vi "UMLEditor Main.vi"(1 "StartProject":string, 3 "StartTarget":string) -> ()   [LabVIEW 2012] (continued)
          n2182 = call-dynamic "getClassInfo.vi"("reference"=w5675, "error in (no error)"=w5689) -> ("reference out"=w5688:refnum<class "ClassNode.lvclass">, "className"=w5685:string, "ClassPath"=w5686:path, "error out"=w5687:errorcluster)  [unwired: 8 in, 6 out]
          n2183 = Select(t=-1, s=w5673, f=w5670) -> (s? t:f=w5672:i32)
          n2184 = Empty String/Path?(string/path=w5686) -> (empty?=w5694:bool)
          n2185 = Not A Number/Path/Refnum?(number/path/refnum=w5686) -> (NaN/Path/Refnum?=w5693:bool)
          n2186 = Or(x=w5694, y=w5693) -> ()  [unwired: 1 out]
          n2187 = Increment(x=w5670) -> (x+1=w5667:i32)
          n2188 = call <resource>:"ReversedEngineering SyncUmlFromCode.vi"("SyncAction"=ReversedEngineering_SyncUmlFromCodeActions."GetAll", "ClassPath"=w5686, "NodeRef"=w5688, "GraphRef"=w5692, "IgnoreClasses"=w5678, "error in (no error)"=w5687, "ClassName(needed for lllbs)"=w5685, "graphics"=w5691, "IterationNo"=w5672, "grid"=w5690, "IterationsN"=w5666) -> ("Cancelled"=w5674:bool, "ClassName"=w5680:string, "attributes"=w5682:string, "methods"=w5681:string, "error out"=w5683:errorcluster)  [unwired: 1 in, 3 out]
          n2189 = Empty String/Path?(string/path=w5680) -> (empty?=w5679:bool)
          n2190 = case shown="False" w5679 {
            tunnel: w5683 -> [w5704 w5709]
            tunnel: w5682 -> [w5703 _]
            tunnel: w5681 -> [w5702 _]
            tunnel: [w5698 w5709] -> w5695
            tunnel: w5688 -> [w5697 _]
            tunnel: w5680 -> [w5696 _]
            frame False {
              n2191 = call-dynamic "ExternalSetParam.vi"("reference"=w5697, "setParameter"=ExternalSetTypes."Attributes", "string"=w5703, "error in (no error)"=w5704) -> ("reference out"=w5706:refnum<class "ClassNode.lvclass">, "error out"=w5707:errorcluster)  [unwired: 14 in]
              n2192 = call-dynamic "ExternalSetParam.vi"("reference"=w5706, "setParameter"=ExternalSetTypes."Methods", "string"=w5702, "error in (no error)"=w5707) -> ("reference out"=w5699:refnum<class "ClassNode.lvclass">, "error out"=w5700:errorcluster)  [unwired: 14 in]
              n2193 = call-dynamic "ExternalSetParam.vi"("reference"=w5699, "setParameter"=ExternalSetTypes."Name", "string"=w5696, "error in (no error)"=w5700) -> ("error out"=w5698:errorcluster)  [unwired: 14 in, 1 out]
            }
            frame True {
            }
          }
          n2194 = Format Into String(format string="Synchronizing %d of %d", w5667, w5666) -> (resulting string=w5668:string)  [unwired: 2 in, 1 out]
          n2195 = local write "StatusBar"(w5668) -> ()
        }
        n2196 = case shown="True" w5635 {
          tunnel: w5634 -> [_ _]
          tunnel: w5632 -> [w5658 w5661]
          tunnel: [w5658 w5660] -> w5631
          frame False {
          }
          frame True {
            n2197 = Get Date/Time In Seconds() -> (seconds since 1Jan1904=w5659:timestamp)
            n2198 = Bundle By Name(cluster=w5661, "LastSync"=w5659) -> (w5660:T7)
            n2199 = property on="Picture" class="Pict"("DisabledEnum"=T38."Enabled" ("Disabled")) -> (error out=w5662:errorcluster)  [unwired: 2 in, 1 out]
            n2200 = call <vilib>:"Unset Busy.vi"("error in (no error)"=w5662) -> ()  [unwired: 10 in, 1 out]
          }
        }
        n2201 = stacked-sequence {
          tunnel: w5634 -> [_]
          tunnel: w5633 -> [w5657]
          frame #0 {
            n2202 = local write "StatusBar"(w5657) -> ()
          }
        }
        n2203 = call <resource>:"UMLEditor setDiagramInfo.vi"("error in (no error)"=w5634, "localVariablesIn"=w5631, "action"=enum16{"Name/Dir", "Unsaved", "Saved"}."Unsaved") -> ("localVariablesOut"=w5646:T7, "error out"=w5648:errorcluster)  [unwired: 2 in, 13 out]
        n2204 = call-dynamic "layout.vi"("reference"=w5642, "error in (no error)"=w5648) -> ("error out"=w5643:errorcluster)  [unwired: 16 in, 1 out]
      }
      frame "StraightenAssociation" {
        n2205 = call <resource>:"UMLEditor getDiagramInfo.vi"("localVariables"=w5727, "error in (no error)"=w5735) -> ("graph"=w5734:refnum<class "Graph.lvclass">, "error out"=w5730:errorcluster)  [unwired: 16 out]
        n2206 = call-dynamic "getEdges.vi"("reference"=w5734, "error in (no error)"=w5730) -> ("reference out"=w5726:refnum<class "Graph.lvclass">, "edges"=w5729:refnum<class "AbstractEdge.lvclass">[], "error out"=w5728:errorcluster)  [unwired: 15 in]
        n2207 = Unbundle By Name(w5727) -> ("graphics"=w5725:refnum<class "Graphics.lvclass">, "grid"=w5724:refnum<class "Grid.lvclass">)
        n2208 = for {
          shift-right: [w5741] -> w5732
          shift-left: w5728 -> [w5744]
          tunnel: w5729 -> [w5743] mode=indexing
          tunnel: w5726 -> [w5739]
          tunnel: w5725 -> [w5738]
          tunnel: w5724 -> [w5737]
          n2209 = call-dynamic "StraightenAssociations.vi"("reference"=w5743, "error in (no error)"=w5744) -> ("reference out"=w5740:refnum<class "AbstractEdge.lvclass">, "error out"=w5742:errorcluster)  [unwired: 16 in]
          n2210 = call-dynamic "Layout.vi"("reference"=w5740, "graph"=w5739, "graphics"=w5738, "grid"=w5737, "error in (no error)"=w5742) -> ("error out"=w5741:errorcluster)  [unwired: 13 in, 1 out]
        }
        n2211 = call <resource>:"UMLEditor setDiagramInfo.vi"("error in (no error)"=w5732, "localVariablesIn"=w5727, "action"=enum16{"Name/Dir", "Unsaved", "Saved"}."Unsaved") -> ("localVariablesOut"=w5731:T7, "error out"=w5723:errorcluster)  [unwired: 2 in, 13 out]
      }
      frame "Exit" {
        # "Check if any unsaved"
        n2212 = Unbundle By Name(w5751) -> ("diagrams"=w5755:T39)
        n2213 = for {
          tunnel: w5755 -> [w5765] mode=indexing
          tunnel: [w5764] -> w5754 mode=indexing
          n2214 = Unbundle By Name(w5765) -> ("unsaved"=w5764:bool)
        }
        n2215 = local read "toolTab"() -> (w5747:enum32{"Class", "Sequence", "UseCase", "State"})
        n2216 = Search 1D Array(1D array=w5754, element=TRUE) -> (index of element=w5750:i32)  [unwired: 1 out]
        n2217 = case shown="\"Class\", Default" w5747 {
          tunnel: [diagramType."Sequency" ("diagramType") diagramType."UseCase" ("diagramType") diagramType."State" ("diagramType") diagramType."Class" ("diagramType")] -> w5746
          frame "Sequence" {
          }
          frame "UseCase" {
          }
          frame "State" {
          }
          frame "Class", Default {
          }
        }
        n2218 = Bundle By Name(cluster=w5751, "quit"=TRUE ("element"), "diagramIndex"=w5750) -> (w5752:T7)
        n2219 = Greater Or Equal To 0?(x=w5750) -> (x >= 0?=w5749:bool)
        n2220 = Select(t=UMLEditor_statesType."Close" ("state"), s=w5749, f=UMLEditor_statesType."QUIT") -> (s? t:f=w5758:T8)
        n2221 = case shown="\"QUIT\"" w5758 {
          tunnel: [w5766 w5769] -> w5759
          tunnel: w5745 -> [w5766 w5773]
          tunnel: w5752 -> [_ w5772]
          tunnel: w5746 -> [_ w5768]
          frame "Idle", Default {
          }
          frame "QUIT" {
            n2222 = call <resource>:"UMLEditor saveIniFileInfo.vi"("localVariables"=w5772, "error in (no error)"=w5773, "diagramType"=w5768) -> ("error out"=w5770:errorcluster)  [unwired: 16 out]
            n2223 = Unbundle By Name(w5770) -> ("code"=w5771:i32)
            n2224 = call <resource>:"UMLEditor_IniFilePath.vi"() -> ("Get Path"=w5767:path)  [unwired: 2 in, 17 out]
            n2225 = case shown="7, 8" w5771 {
              tunnel: w5770 -> [w5774 _]
              tunnel: [w5774 errorcluster {"status"=FALSE, "code"=0, "source"=""} ("error out")] -> w5769
              tunnel: w5767 -> [_ w5775]
              frame 0, Default {
              }
              frame 7, 8 {
                n2226 = Format Into String(format string="File permission error.\n\nMake sure the file to modify is writable.\n%s" ("message"), w5775) -> (resulting string=w5777:string)  [unwired: 2 in, 1 out]
                n2227 = One Button Dialog(message=w5777) -> ()  [unwired: 2 out]
              }
            }
          }
        }
      }
      frame "Error", Default {
        n2228 = Format Into String(w5782) -> (resulting string=w5781:string)  [unwired: 3 in, 1 out]
        n2229 = Unbundle By Name(w5779) -> ("code"=w5784:i32)
        n2230 = case shown="1055" w5784 {
          tunnel: [TRUE ("s") FALSE ("s") FALSE ("s") FALSE ("s") FALSE ("s") FALSE ("s") FALSE ("s") FALSE ("s") FALSE ("s") _ FALSE ("s")] -> w5783
          tunnel: w5781 -> [w5791 _ _ _ _ _ _ _ _ _ _]
          tunnel: w5780 -> [w5790 _ _ _ _ _ _ _ _ _ _]
          tunnel: w5779 -> [_ _ _ _ _ _ _ _ _ w5809 _]
          frame 0, Default {
            n2231 = call <resource>:"GDSError_LogErrorInformation.vi"("State"=w5791, "LocalVariableData"=w5790) -> ()  [unwired: 2 in, 16 out]
          }
          frame 1106, 1108 {
            n2232 = One Button Dialog(message="The saved file you tried to open,\nwas not compatible with this version.") -> ()  [unwired: 2 out]
          }
          frame 1044 {
            n2233 = One Button Dialog(message="A VI was locked, so the task has been stopped.") -> ()  [unwired: 2 out]
          }
          frame 1073 {
            n2234 = One Button Dialog(message="Trying to access a write protected file, or\na file that is currently running or reserved\nfor execution.") -> ()  [unwired: 2 out]
          }
          frame 56003 {
            n2235 = One Button Dialog(message="The new class(es) could not be added to the project since it would cause a conflict with an item already in memory.\n-This could be due to that the class created already exists in another opened project. Try to close other none used project to prevent this from happening.") -> ()  [unwired: 2 out]
          }
          frame 1025 {
            n2236 = One Button Dialog(message="The project reference is invalid.\nMake sure you have a selected project.") -> ()  [unwired: 2 out]
          }
          frame 1055 {
            n2237 = One Button Dialog(message="Class/Project reference error.\nThe reason for this could be:\n-The project has been closed\n-The class(es) has been removed from the project\n-The class(es) don't exist in the selected project") -> ()  [unwired: 2 out]
          }
          frame 7000 {
            n2238 = One Button Dialog(message="The class reference could not be obtained from the project.\nThe reason for this could be:\n-The project has been closed\n-The class has been removed from the project\n-The class don't exist in the selected project") -> ()  [unwired: 2 out]
          }
          frame 56001 {
            n2239 = One Button Dialog(message="Class(es) with the same name already exists in the project.") -> ()  [unwired: 2 out]
          }
          frame 5011 {
            n2240 = call <resource>:"GDSError_ReportError.vi"("error in (no error)"=w5809) -> ()  [unwired: 19 out]
          }
          frame 8 {
            n2241 = One Button Dialog(message="File permission error.\n\nMake sure the file to modify is writable.") -> ()  [unwired: 2 out]
          }
        }
        n2242 = Select(t=w5779, s=w5783, f=errorcluster {"status"=FALSE, "code"=0, "source"=""} ("error out")) -> (s? t:f=w5785:errorcluster)
        n2243 = Select(t=UMLEditor_statesType."QUIT" ("state"), s=w5783, f=UMLEditor_statesType."Idle" ("state")) -> (s? t:f=w5789:T8)
      }
    }
    n2244 = Select(t=UMLEditor_statesType."Error" ("state"), s=w32, f=w37) -> (s? t:f=w38:T8)
    n2245 = case shown="Error" w32 {
      frame No Error {
      }
      frame Error {
      }
    }
    n2246 = Equal?(x=w37, y=UMLEditor_statesType."QUIT" ("state")) -> (x = y?=w45:bool)
  }
  n2247 = Unbundle By Name(w9) -> ("graphics"=w24:refnum<class "Graphics.lvclass">, "grid"=w26:refnum<class "Grid.lvclass">, "diagrams"=w22:T39)
  n2248 = for {
    shift-right: [w5813] -> w23
    shift-left: w5 -> [w5814]
    tunnel: w22 -> [w5815] mode=indexing
    n2249 = Unbundle By Name(w5815) -> ("graph"=w5812:refnum<class "Graph.lvclass">)
    n2250 = call-dynamic "Destroy.vi"("reference"=w5812, "error in (no error)"=w5814) -> ("error out"=w5813:errorcluster)  [unwired: 16 in, 1 out]
  }
  n2251 = call-dynamic "Destroy.vi"("reference"=w26, "error in (no error)"=w23) -> ("error out"=w25:errorcluster)  [unwired: 16 in, 1 out]
  n2252 = call-dynamic "Destroy.vi"("reference"=w24, "error in (no error)"=w25) -> ("# of objects"=w12:i32)  [unwired: 16 in, 1 out]
  n2253 = case shown="Error" w5 {
    selector: w5 -> [w5816 w5817]
    tunnel: [w5816 w5817] -> w20
    tunnel: w9 -> [_ _]
    tunnel: w12 -> [_ _]
    frame No Error {
    }
    frame Error {
      n2254 = call <resource>:"GDSError_ReportError.vi"("error in (no error)"=w5817) -> ()  [unwired: 19 out]
    }
  }
  n2255 = Unbundle By Name(w9) -> ("Cursors"=w4:refnum<k1>[])
  n2256 = Unbundle By Name(w9) -> ("Event"=w8:refnum<event-registration>, "ViRef"=w19:refnum<vi>)
  n2257 = Close Reference(reference=w19, error in (no error)=w20) -> (error out=w17:errorcluster)
  n2258 = stacked-sequence {
    tunnel: w17 -> [w5826]
    tunnel: [w5826] -> w16
    tunnel: w8 -> [w5819]
    tunnel: w4 -> [w5818]
    frame #0 {
      # "Kill Tasks"
      n2259 = call <resource>:"ContextHelp_StopPopUpTask.vi"() -> ()  [unwired: 2 in, 18 out]
      n2260 = call <resource>:"UMLEditor ClipBoard.vi"("menuAction"=UMLEditor_ClipBoardActionType."EmptyClipBoard") -> ()  [unwired: 5 in, 14 out]
      n2261 = call <resource>:"CleanUp.vi"() -> ()  [unwired: 1 in, 19 out]
      n2262 = call <resource>:"UMLEditor ControlBusyDialog.vi"("Action(SendStatusMessage)"=UMLEditor_BusyDialogAction."Quit" ("Action")) -> ()  [unwired: 3 in, 16 out]
      n2263 = for {
        tunnel: w5818 -> [w5827] mode=indexing
        n2264 = call <vilib>:"Destroy Cursor.vi"("cursor ID"=w5827) -> ()  [unwired: 1 in, 9 out]
      }
      n2265 = call <resource>:"CommonVIs_UmlOpenVIRef.vi"("ProjectNameIn"="clear" ("pattern (all files)")) -> ()  [unwired: 3 in, 8 out]
      n2266 = Unregister For Events(event registration refnum=w5819) -> ()  [unwired: 1 in, 1 out]
      n2267 = property on="SearchString" class="Str"("Visible"=FALSE, "Value"="" ("SearchString")) -> ()  [unwired: 2 in, 2 out]
      n2268 = call <resource>:"GOOP_MouseFunctions.vi"("Action(Read)"=enum16{"Init", "Read", "Close"}."Close") -> ()  [unwired: 8 in, 3 out]
    }
  }
  n2269 = call <resource>:"UMLEditor RemoveStaticObjects.vi"("error in (no error)"=w16) -> ("error out"=w18:errorcluster)  [unwired: 18 out]
  "error out" <- w18
  n2270 = property on="Time" class="DigNum (strict)"("Visible"=w1) -> ()  [unwired: 2 in, 2 out]
  n2271 = disable-structure shown="Disabled" {
    disable-tunnel: w18 -> [w5830 _]
    disable-tunnel: w7 -> [w5829 _]
    disable-tunnel: w1 -> [w5828 _]
    frame Disabled {
      n2272 = stacked-sequence {
        tunnel: w5828 -> [_]
        tunnel: w5830 -> [_]
        tunnel: w5829 -> [w5833]
        tunnel: [w5832] -> _
        frame #0 {
          n2273 = invoke class="VI" method="FP.Close"(reference=w5833) -> (reference out=w5834:refnum<vi>, error out=w5835:errorcluster)  [unwired: 2 in, 1 out]
          n2274 = property on="Time" class="DigNum (strict)"("Visible"=FALSE) -> ()  [unwired: 2 in, 2 out]
          n2275 = Close Reference(reference=w5834, error in (no error)=w5835) -> (error out=w5832:errorcluster)
        }
      }
    }
    frame Enabled {
    }
  }
